vi "Project_1.vi"() -> ()   [LabVIEW 2020]
uses:
  <vilib>/Utility/file.llb/Read Delimited Spreadsheet (string).vi
  <vilib>/Utility/file.llb/Read Delimited Spreadsheet (DBL).vi
panel:
  in  "要從第幾行\n開始看":dbl(slide) scale=0.0..1800.0
  out "資料標題":string
  out "Waveform Graph":dbl[](graph)
  in  "stop":bool
  out "列表部分Y值":dbl[](array[numeric])
  in  "想看的列  (col)":i32
  in  "資料路徑":path
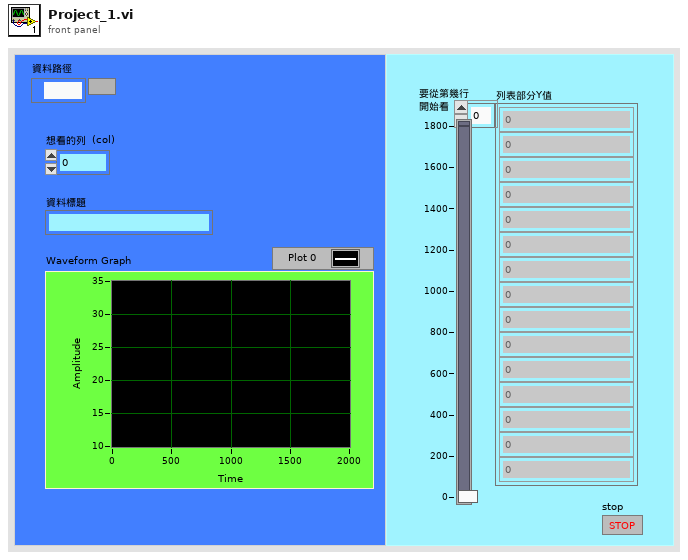
[diagram p1: front panel]
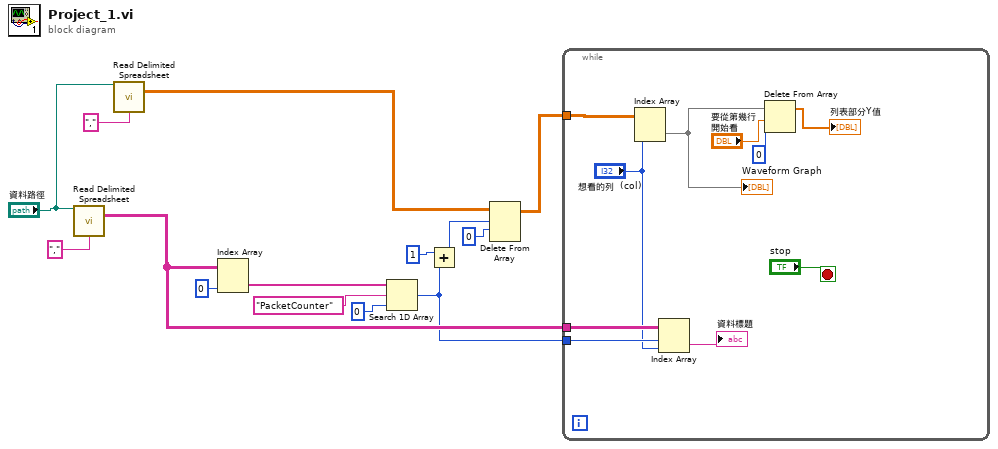
[diagram p0: block diagram]
diagram:
  n1 = call-poly <vilib>:"Read Delimited Spreadsheet.vi"("file path (dialog if empty)"="資料路徑", "delimiter (\\t)"="," ("delimiter (\\t)")) -> ("all rows"=w2:string[][])  [unwired: 8 in, 5 out]
  n2 = call-poly <vilib>:"Read Delimited Spreadsheet.vi"("file path (dialog if empty)"="資料路徑", "delimiter (\\t)"="," ("delimiter (\\t)")) -> ("all rows"=w4:dbl[][])  [unwired: 8 in, 5 out]
  n3 = Index Array(array=w2, index (col)=0 ("disabled index (col)")) -> (element=w12:string[])  [unwired: 1 in]
  n4 = Search 1D Array(1D array=w12, element="PacketCounter", start index (0)=0) -> (index of element=w1:i32)
  n5 = Add(x=1, y=w1) -> (x+y=w8:i32)
  n6 = Delete From Array(array=w4, length=w8, index (row)=0 ("index")) -> (array with subset deleted=w6:dbl[][])  [unwired: 1 in, 1 out]
  n7 = while {
    tunnel: w6 -> [w24]
    tunnel: w2 -> [w22]
    tunnel: w1 -> [w21]
    stop <- "stop" stop-if-true
    n8 = Index Array(array=w24, index (col)="想看的列  (col)") -> (element=w18:dbl[])  [unwired: 1 in]
    "Waveform Graph" <- w18
    n9 = Index Array(array=w22, index (row)=w21, index (col)="想看的列  (col)") -> (element=→"資料標題":string)
    n10 = Delete From Array(array=w18, length="要從第幾行\n開始看", index=0) -> (array with subset deleted=→"列表部分Y值":dbl[])  [unwired: 1 out]
  }
